vi "shiftOutsideDistanceFromQuad.vi"(8 "error in (no error)":errorcluster, 9 "Pos de Interseção":dbl[](array[numeric]) format="%#_13g", 10 "Game":refnum<class "Game.lvclass">, 11 "Utilities in":refnum<class "Utilities.lvclass">) -> (0 "error out":errorcluster, 2 "Array":dbl[](array[numeric]), 3 "Utilities out":refnum<class "Utilities.lvclass">)   [LabVIEW 2023, in "Utilities.lvclass"]
uses:
  Utilities.lvclass
  Game_class/Game.lvclass
  Game_class/Game.lvclass/Game.ctl
  Game_class/Read FieldRef.vi
  Game_class/Read Parameters.lvclass.vi
  Field_class/Field.lvclass
  Parameters_class/Parameters.lvclass
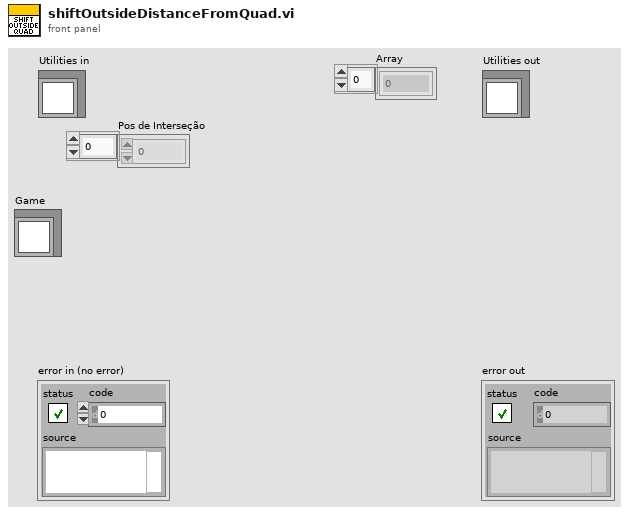
[diagram p1: front panel]
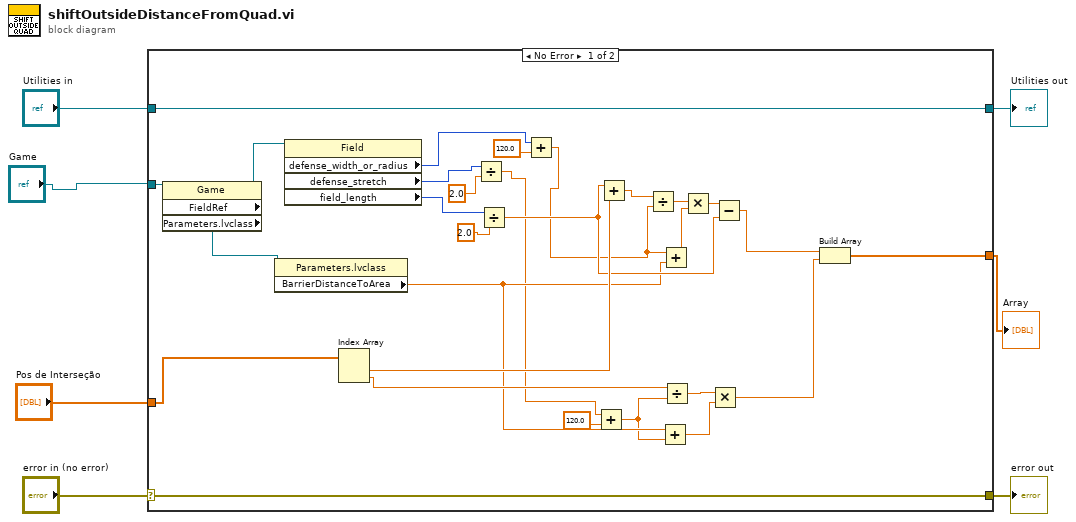
[diagram p0: block diagram]
diagram:
  n1 = case shown="No Error" "error in (no error)" {
    selector: "error in (no error)" -> [w35 w38]
    tunnel: [w35 w38] -> w6
    tunnel: [w36 w37] -> w4
    tunnel: "Utilities in" -> [w36 w37]
    tunnel: "Game" -> [w34 _]
    tunnel: "Pos de Interseção" -> [w31 _]
    tunnel: [w16 _] -> w1
    frame No Error {
      n2 = property class="Game"(reference=w34) -> ("FieldRef"=w33:refnum<class "Field.lvclass">, "Parameters.lvclass"=w32:refnum<class "Parameters.lvclass">)  [unwired: 1 in, 2 out]
      n3 = property class="Parameters.lvclass"(reference=w32) -> ("BarrierDistanceToArea"=w18:dbl)  [unwired: 1 in, 2 out]
      n4 = property class="Field"(reference=w33) -> ("defense_width_or_radius"=w13:i32, "defense_stretch"=w15:i32, "field_length"=w29:i32)  [unwired: 1 in, 2 out]
      n5 = Index Array(array=w31) -> (element #1=w28:dbl, element #2=w21:dbl)  [unwired: 2 in]
      n6 = Divide(x=w15, y=2.0) -> (x/y=w9:dbl)
      n7 = Divide(x=w29, y=2.0) -> (x/y=w23:dbl)
      n8 = Add(x=w13, y=120.0) -> (x+y=w11:dbl)
      n9 = Add(x=w9, y=120.0) -> (x+y=w8:dbl)
      n10 = Add(x=w23, y=w28) -> (x+y=w27:dbl)
      n11 = Divide(x=w27, y=w11) -> (x/y=w26:dbl)
      n12 = Add(x=w18, y=w8) -> (x+y=w19:dbl)
      n13 = Add(x=w11, y=w18) -> (x+y=w25:dbl)
      n14 = Divide(x=w21, y=w8) -> (x/y=w20:dbl)
      n15 = Multiply(x=w26, y=w25) -> (x*y=w24:dbl)
      n16 = Multiply(x=w20, y=w19) -> (x*y=w17:dbl)
      n17 = Subtract(x=w24, y=w23) -> (x-y=w22:dbl)
      n18 = Build Array(w22, w17) -> (w16:dbl[])
    }
    frame Error {
    }
  }
  "error out" <- w6
  "Utilities out" <- w4
  "Array" <- w1
